vi "Selected Range Query.vi"(8 "error in (no error)":errorcluster, 10 "Function":string(combo)="VOLT", 11 "VISA resource name":refnum<visa-resource-name>="GPIB0::24::INSTR") -> (0 "error out":errorcluster, 2 "Selected Range":dbl format="%_1e", 3 "VISA resource name out":refnum<visa-resource-name>)   [LabVIEW 2022 SP3, in "Keithley 2450.lvlib"]
doc: "This VI returns the active range for the selected function on the 2450 SMU."
uses:
  Keithley 2450.lvlib
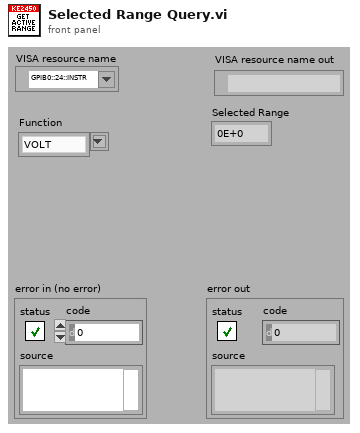
[diagram p1: front panel]
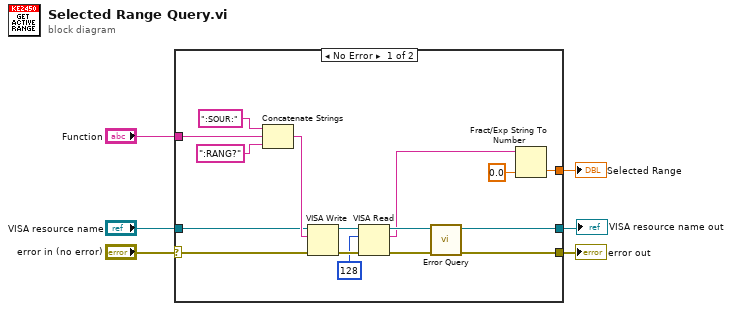
[diagram p0: block diagram]
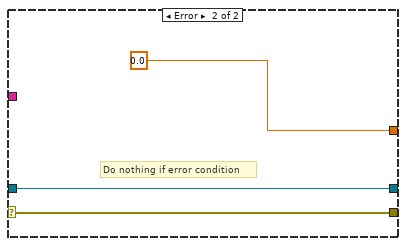
[diagram p2: hidden frame]
diagram:
  n1 = case shown="No Error" "error in (no error)" {
    selector: "error in (no error)" -> [w9 w25]
    tunnel: [w22 w25] -> w5
    tunnel: "VISA resource name" -> [w10 w24]
    tunnel: [w21 w24] -> w1
    tunnel: [w8 0.0] -> w3
    tunnel: "Function" -> [w12 _]
    frame No Error {
      n2 = Concatenate Strings(":SOUR:" ("string"), w12, ":RANG?" ("string")) -> (w14:string)
      n3 = VISA Write(VISA resource name=w10, write buffer=w14, error in (no error)=w9) -> (VISA resource name out=w18:refnum<visa-resource-name>, error out=w19:errorcluster)  [unwired: 1 out]
      n4 = VISA Read(VISA resource name=w18, byte count=u32 128, error in (no error)=w19) -> (VISA resource name out=w16:refnum<visa-resource-name>, read buffer=w7:string, error out=w17:errorcluster)  [unwired: 1 out]
      n5 = call "Error Query.vi"("error in (no error)"=w17, "VISA resource name"=w16) -> ("error out"=w22:errorcluster, "VISA resource name out"=w21:refnum<visa-resource-name>)  [unwired: 8 out]
      n6 = Fract/Exp String To Number(string=w7, default (0 dbl)=0.0 ("default (0 I32)")) -> (number=w8:dbl)  [unwired: 3 out]
    }
    frame Error {
      # "Do nothing if error condition"
    }
  }
  "error out" <- w5
  "Selected Range" <- w3
  "VISA resource name out" <- w1
